vi "CreatePrivateEvents.vi"(8 "error in (no error)":errorcluster, 11 "Generator":refnum<class "Generator.lvclass">) -> (0 "error out":errorcluster, 3 "Generator out":refnum<class "Generator.lvclass">)   [LabVIEW 2019, in "Generator.lvclass"]
uses:
  Generator.lvclass
  typedefs/Message--Cluster.ctl
  Generator.lvclass/Generator.ctl
  <vilib>/JKI/JKI SMO/SMO/SMO.lvclass
panel:
  # "For instructions on how to use the JKI State Machine Objects, examples and video tutorials, visit:\nhttp://jki.net/state-machine-objects/\n\nJKI State Machine Objects™\nhttp://jki.net/state-machine-objects/\nCopyright (C) 2005-2015, JKI <info@jki.net>\nALL RIGHTS RESERVED"
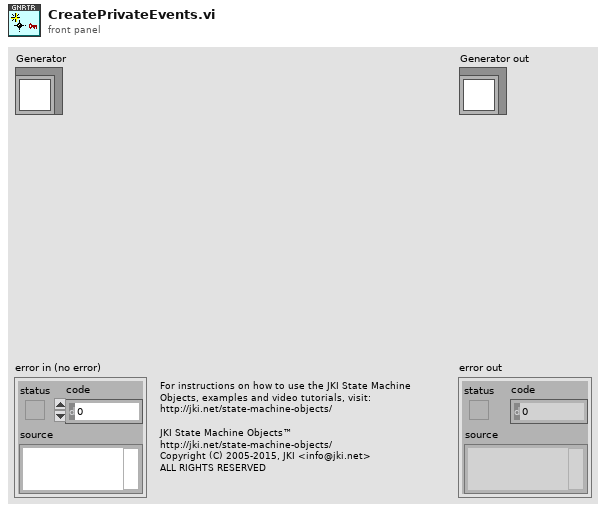
[diagram p1: front panel]
types:
  T1 = typedef "Generator.lvclass/Message--Cluster.ctl" = cluster{"Command":string, "Data":variant}
  T2 = typedef "Generator.lvclass/AO.Channel--Cluster--Array.ctl" = T3[]
  T3 = typedef "Generator.lvclass/AO.Channel--Cluster.ctl" = cluster{"Enable?":bool, "Channel":i32, "Amplitude":dbl, "Offset":dbl, "Frequency":dbl, "Phase":dbl, "Function":T4, "Sweeping?":bool, "Limit AC":bool, "Limit DC?":bool}
  T4 = typedef "Generator.lvclass/AO.Channel.Function--Enum.ctl" = enum16{"Sine", "Triangle", "Square"}
  T5 = cluster{"Enable?":bool, "Channel":i32, "Frequency":dbl, "Phase":dbl, "TC":dbl, "Roll-Off":i32}[]
  T6 = typedef "Generator.lvclass/Sweep.Configuration--Cluster.ctl" = cluster{"Sweep Time (s)":dbl, "Initial Wait (s)":dbl, "Return to Start":bool, "Channels":T7}
  T7 = typedef "Generator.lvclass/Sweep.Channel--Cluster--Array.ctl" = T8[]
  T8 = typedef "Generator.lvclass/Sweep.Channel--Cluster.ctl" = cluster{"Enable?":bool, "Channel":u16, "Start":dbl, "End":dbl, "Pattern":T9, "Table":dbl[]}
  T9 = typedef "Generator.lvclass/Sweep.Pattern--Enum.ctl" = enum16{"Ramp /", "Ramp /\\", "Smooth Ramp _/", "Smooth Ramp _/\\_", "Table"}
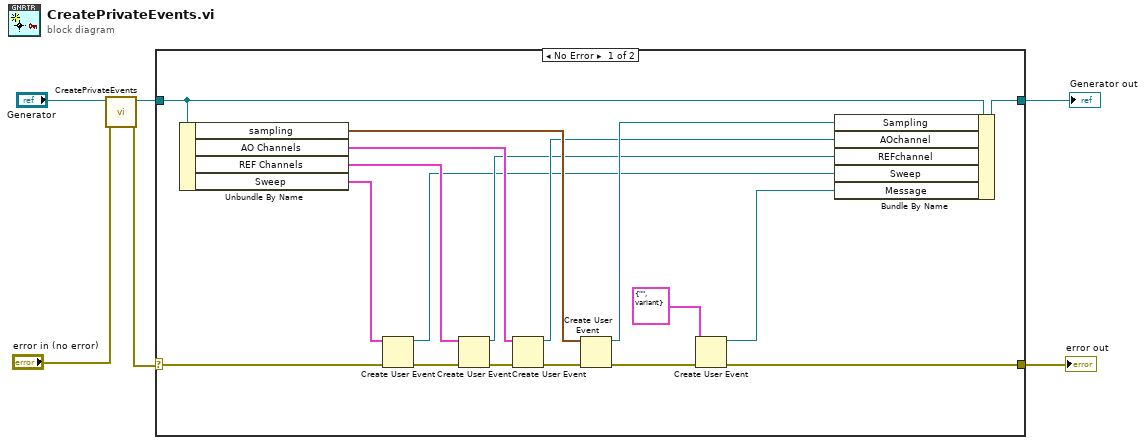
[diagram p0: block diagram]
diagram:
  n1 = call-parent "CreatePrivateEvents.vi"("error in (no error)"="error in (no error)", "SMO"="Generator") -> ("error out"=w4:errorcluster, "SMO out"=w5:refnum<class "Generator.lvclass">)  [unwired: 8 in]
  n2 = case shown="No Error" w4 {
    selector: w4 -> [w20 w26]
    tunnel: [w8 w26] -> w2
    tunnel: [w24 w25] -> w3
    tunnel: w5 -> [w23 w25]
    frame No Error {
      n3 = Unbundle By Name(w23) -> ("sampling"=w15:cluster{"Fs":dbl, "#s":dbl}, "AO Channels"=w16:T2, "REF Channels"=w17:T5, "Sweep"=w18:T6)
      n4 = Create User Event(user event datatype=w18, error in=w20) -> (user event=w10:refnum<user-event>, error out=w21:errorcluster)
      n5 = Create User Event(user event datatype=w17, error in=w21) -> (user event=w11:refnum<user-event>, error out=w19:errorcluster)
      n6 = Create User Event(user event datatype=w16, error in=w19) -> (user event=w12:refnum<user-event>, error out=w22:errorcluster)
      n7 = Create User Event(user event datatype=w15, error in=w22) -> (user event=w13:refnum<user-event>, error out=w14:errorcluster)
      n8 = Create User Event(user event datatype=T1 {"Command"="", "Data"=variant} ("Message"), error in=w14) -> (user event=w9:refnum<user-event>, error out=w8:errorcluster)
      n9 = Bundle By Name(cluster=w23, "Sampling"=w13, "AOchannel"=w12, "REFchannel"=w11, "Sweep"=w10, "Message"=w9) -> (w24:refnum<class "Generator.lvclass">)
    }
    frame Error {
    }
  }
  "error out" <- w2
  "Generator out" <- w3
